vi "Status Test.vi"() -> ()   [LabVIEW 2014, in "ESP8266 WiFi Wrapper.lvlib"]
uses:
  ESP8266 WiFi Wrapper.lvlib
panel:
  out "Status":u8(ring) items=["WL_NO_SHIELD"=255, "WL_IDLE_STATUS"=0, "WL_NO_SSID_AVAIL"=1, "WL_SCAN_COMPLETED"=2, "WL_CONNECTED"=3, "WL_CONNECT_FAILED"=4, "WL_CONNECTION_LOST"=5, "WL_DISCONNECTED"=6]
  out "Error Out":errorcluster
  in  "Error In":errorcluster
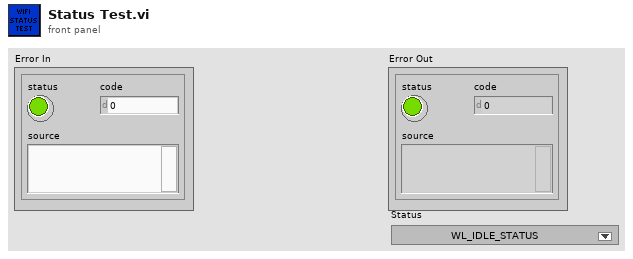
[diagram p1: front panel]
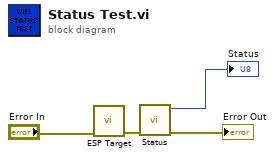
[diagram p0: block diagram]
diagram:
  n1 = call "ESP Target.vi"("Error In"="Error In") -> ("Error Out"=w2:errorcluster)  [unwired: 10 in]
  n2 = call "Status.vi"("Error In"=w2) -> ("Error Out"=→"Error Out":errorcluster, "Status"=→"Status":u8)  [unwired: 9 in]
